vi "Introspection Core.vi"(8 "error in (no error)":errorcluster, 11 "CS++DSCMonitor in":refnum<class "CS++DSCMonitor.lvclass">) -> (0 "error out":errorcluster, 2 "CS++Messages":refnum<class "Message.lvclass">[](array[class]), 3 "CS++DSCMonitor out":refnum<class "CS++DSCMonitor.lvclass">)   [LabVIEW 2014, in "CS++DSCMonitor.lvlib" / "CS++DSCMonitor.lvclass"]
doc: "This vi delivers a list with all messages this actor reacts to. \n\nNote that all inherited classes have to overwrite it."
uses:
  CS++DSCMonitor.lvclass
  CSPP_Core/Actors/CS++SVMonitor/CS++SVMonitor.lvclass
  <vilib>/ActorFramework/Message/Message.lvclass
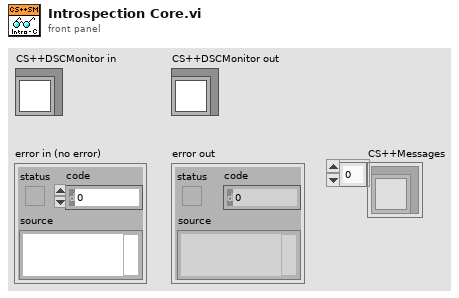
[diagram p1: front panel]
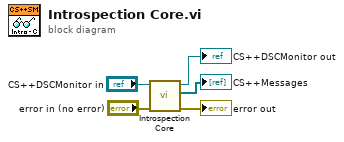
[diagram p0: block diagram]
diagram:
  n1 = call-parent "Introspection Core.vi"("error in (no error)"="error in (no error)", "CS++SVMonitor in"="CS++DSCMonitor in") -> ("error out"=→"error out":errorcluster, "CS++Messages"=→"CS++Messages":refnum<class "Message.lvclass">[], "CS++SVMonitor out"=→"CS++DSCMonitor out":refnum<class "CS++DSCMonitor.lvclass">)  [unwired: 7 in]
